vi "dequeueMessage.vi"(8 "error in (no error)":errorcluster) -> (0 "error out":errorcluster, 3 "element":T1)   [LabVIEW 2017, in "programControl.lvlib"]
uses:
  programControl.lvlib
  TypeDefs/message.ctl
  TypeDefs/queueFGVState.ctl
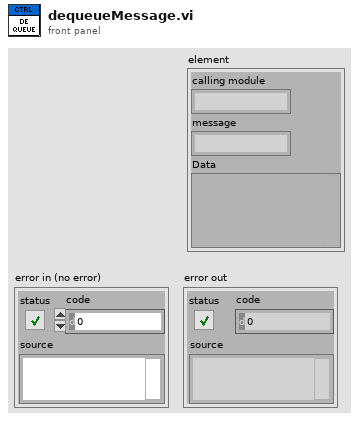
[diagram p1: front panel]
types:
  T1 = typedef "programControl.lvlib/message.ctl" = cluster{"calling module":string, "message":string, "Data":variant}
  T2 = typedef "programControl.lvlib/queueFGVState.ctl" = enum16{"get", "set"}
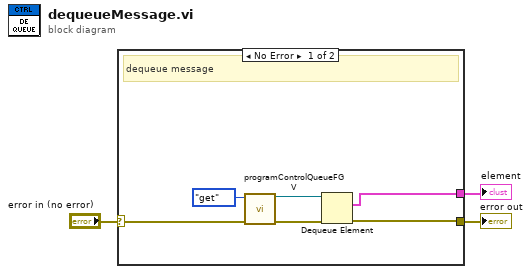
[diagram p0: block diagram]
diagram:
  n1 = case shown="No Error" "error in (no error)" {
    selector: "error in (no error)" -> [w8 w10]
    tunnel: [w6 w10] -> w2
    tunnel: [w4 _] -> w1
    frame No Error {
      # "dequeue message"
      n2 = call "programControlQueueFGV.vi"("error in (no error)"=w8, 11:queueFGVState."get") -> ("error out"=w7:errorcluster, "queue out"=w5:refnum<queue>)  [unwired: 8 in]
      n3 = Dequeue Element(queue=w5, error in (no error)=w7) -> (element=w4:T1, error out=w6:errorcluster)  [unwired: 1 in, 2 out]
    }
    frame Error {
    }
  }
  "error out" <- w2
  "element" <- w1
